vi "Get Test Method Result.vi"(11 "LUnit Test Case In":refnum<class "LUnit Test Case.lvclass">) -> (2 "Test Method Result":T1, 3 "LUnit Test Case Out":refnum<class "LUnit Test Case.lvclass">)   [LabVIEW 2020, in "LUnit Test Case.lvclass"]
uses:
  LUnit Test Case.lvclass
  Result Types/Method Result/Method Result.ctl
  Result Types/Assertion Result/Public/TypeDefs/Status.ctl
  Result Types/Assertion Result/Assertion Result.ctl
  Result Types/Assertion Result/Public/TypeDefs/Assertion Type.ctl
  LUnit Test Case.lvclass/LUnit Test Case.ctl
  Result Types/Case Result/Test Case Result.lvlib
  Result Types/Assertion Result/Assertion Result.lvlib
  Result Types/Method Result/Method Result.lvlib
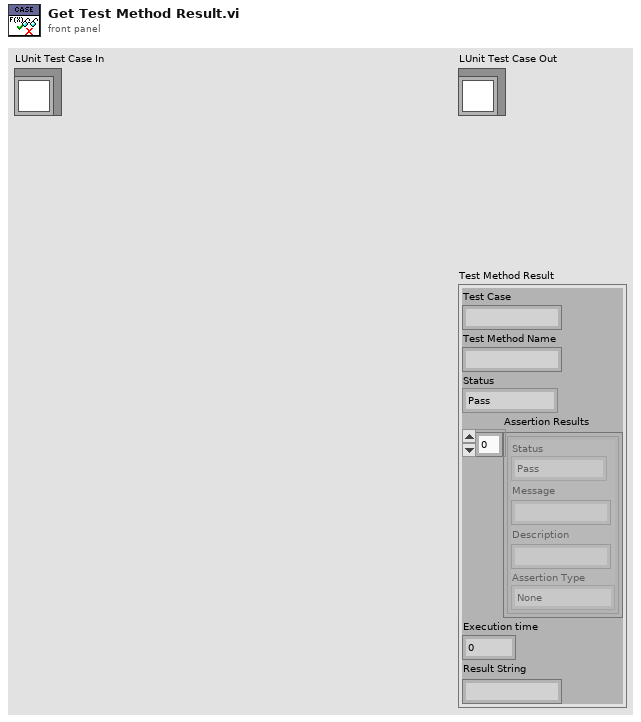
[diagram p1: front panel]
types:
  T1 = typedef "Method Result.lvlib/Method Result.ctl" = cluster{"Test Case":string, "Test Method Name":string, "Status":T2, "Assertion Results":T3[], "Execution time":dbl, "Result String":string}
  T2 = typedef "Assertion Result.lvlib/Status.ctl" = enum16{"Pass", "Fail", "Error", "Skipped", "Setup Error", "Broken", "Teardown Error"}
  T3 = typedef "Assertion Result.lvlib/Assertion Result.ctl" = cluster{"Status":T2, "Message":string, "Description":string, "Assertion Type":T4}
  T4 = typedef "Assertion Result.lvlib/Assertion Type.ctl" = enum16{"None", "Pass", "Fail", "Skip", "Pass if Equal", "Fail if Equal", "Pass if Error", "Fail if Error", "Pass if", "Fail if"}
  T5 = typedef "Test Case Result.lvlib/Test Case Result.ctl" = map{string, T1}
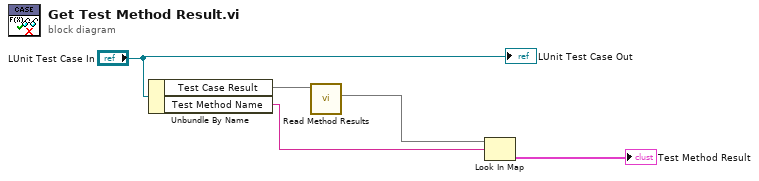
[diagram p0: block diagram]
diagram:
  n1 = Unbundle By Name("LUnit Test Case In") -> ("Test Case Result"=w2:T5, "Test Method Name"=w5:string)
  n2 = call "Read Method Results.vi"("Test Case Result In"=w2) -> ("Method Results"=w1:map{string, T1})  [unwired: 9 in, 1 out]
  n3 = Look In Map(map=w1, key=w5) -> (value=→"Test Method Result":T1)  [unwired: 1 in, 1 out]
  "LUnit Test Case Out" <- "LUnit Test Case In"
